vi "reset.vi"(10 "up/down in":T2, 11 "floor cluster in":T1) -> (2 "up/down out":T2, 3 "floor cluster out":T1)   [LabVIEW 2020]
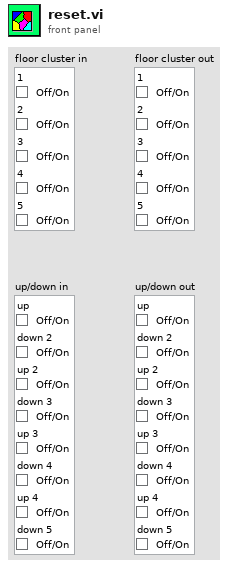
[diagram p1: front panel]
types:
  T1 = cluster{"1":bool, "2":bool, "3":bool, "4":bool, "5":bool}
  T2 = cluster{"up":bool, "down 2":bool, "up 2":bool, "down 3":bool, "up 3":bool, "down 4":bool, "up 4":bool, "down 5":bool}
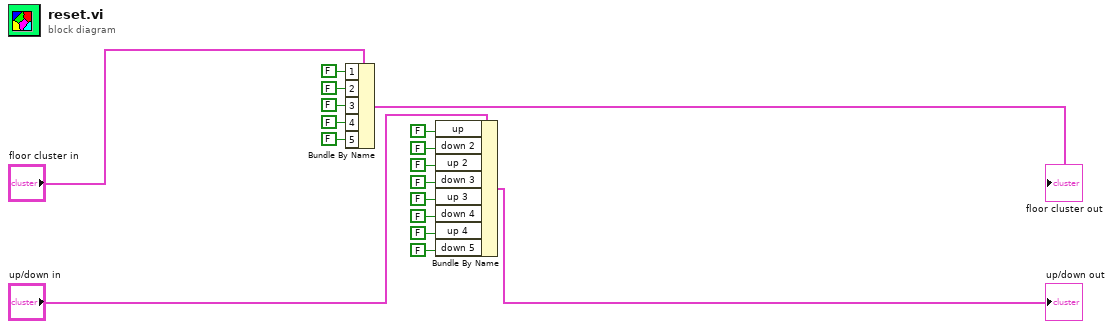
[diagram p0: block diagram]
diagram:
  n1 = Bundle By Name(cluster="floor cluster in", "1"=FALSE, "2"=FALSE, "3"=FALSE, "4"=FALSE, "5"=FALSE) -> (→"floor cluster out":T1)
  n2 = Bundle By Name(cluster="up/down in", "up"=FALSE, "down 2"=FALSE, "up 2"=FALSE, "down 3"=FALSE, "up 3"=FALSE, "down 4"=FALSE, "up 4"=FALSE, "down 5"=FALSE) -> (→"up/down out":T2)
